vi "TestTranslateVI.vi"(8 "error in (no error)":errorcluster) -> (0 "error out":errorcluster)   [LabVIEW 2017]
uses:
  <vilib>/addons/_JKI Toolkits/Caraya/classes/Test/Test.lvclass
  src/API/JKI Simple Localization.lvlib
  <vilib>/addons/_JKI Toolkits/Caraya/classes/Assert/Assert.lvclass
panel:
  # "See block diagram for unit tests of TranslateVI.vi"
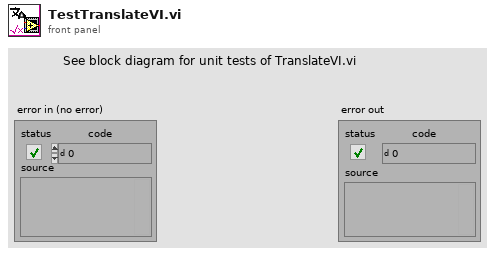
[diagram p1: front panel]
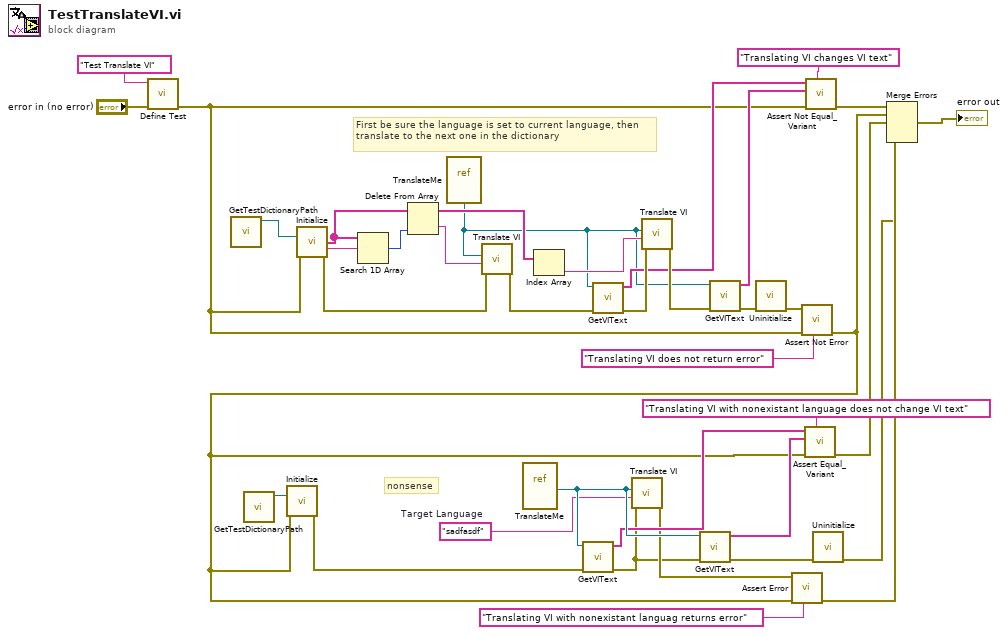
[diagram p0: block diagram]
diagram:
  w22 = "sadfasdf"  # Target Language
  # "nonsense"
  # "First be sure the language is set to current language, then translate to the next one in the dictionary"
  n1 = call <vilib>:"Define Test.vi"("error in (no error)"="error in (no error)", "Label (VI Title)"="Test Translate VI") -> ("error out"=w19:errorcluster)  [unwired: 9 in]
  n2 = call "GetTestDictionaryPath.vi"() -> ("Test Dictionary Path"=w36:path)  [unwired: 11 in]
  n3 = call "GetTestDictionaryPath.vi"() -> ("Test Dictionary Path"=w21:path)  [unwired: 11 in]
  n4 = call "Initialize.vi"("Dictionary File Path"=w36, "error in"=w19) -> ("Languages"=w30:string[], "Current Language"=w11:string, "error out"=w8:errorcluster)  [unwired: 10 in, 1 out]
  n5 = Search 1D Array(1D array=w30, element=w11) -> (index of element=w31:i32)  [unwired: 1 in]
  n6 = Delete From Array(array=w30, index=w31) -> (deleted portion=w9:string, array with subset deleted=w13:string[])  [unwired: 1 in]
  n7 = vi-ref "TranslateMe.vi"() -> (w10:refnum<vi>)
  n8 = call "Translate VI.vi"("error in"=w8, "Target Language"=w9, "VI Ref"=w10) -> ("error out"=w7:errorcluster)  [unwired: 8 in]
  n9 = vi-ref "TranslateMe.vi"() -> (w24:refnum<vi>)
  n10 = Index Array(array=w13) -> (element=w12:string)  [unwired: 1 in]
  n11 = call "GetVIText.vi"("error in (no error)"=w7, "VI"=w10) -> ("error out"=w29:errorcluster, "Control Text"=w26:string[])  [unwired: 7 in, 1 out]
  n12 = call "Translate VI.vi"("error in"=w29, "Target Language"=w12, "VI Ref"=w10) -> ("error out"=w28:errorcluster)  [unwired: 8 in]
  n13 = call "GetVIText.vi"("error in (no error)"=w28, "VI"=w10) -> ("error out"=w27:errorcluster, "Control Text"=w25:string[])  [unwired: 7 in, 1 out]
  n14 = call "Uninitialize.vi"("error in"=w27) -> ("error out"=w2:errorcluster)  [unwired: 10 in]
  n15 = call <vilib>:"Assert Not Error.vi"("Label"="Translating VI does not return error", "error in (no error)"=w19, "Not Error?"=w2) -> ("error out"=w16:errorcluster)  [unwired: 8 in]
  n16 = call "Initialize.vi"("Dictionary File Path"=w21, "error in"=w16) -> ("error out"=w23:errorcluster)  [unwired: 10 in, 3 out]
  n17 = call "GetVIText.vi"("error in (no error)"=w23, "VI"=w24) -> ("error out"=w5:errorcluster, "Control Text"=w17:string[])  [unwired: 7 in, 1 out]
  n18 = call "Translate VI.vi"("error in"=w5, "Target Language"=w22, "VI Ref"=w24) -> ("error out"=w6:errorcluster)  [unwired: 8 in]
  n19 = call "GetVIText.vi"("error in (no error)"=w5, "VI"=w24) -> ("error out"=w4:errorcluster, "Control Text"=w18:string[])  [unwired: 7 in, 1 out]
  n20 = call <vilib>:"Assert Error.vi"("Label"="Translating VI with nonexistant languag returns error", "error in (no error)"=w16, "Error?"=w6) -> ("error out"=w3:errorcluster)  [unwired: 8 in]
  n21 = call <vilib>:"Assert Equal_Variant.vi"("Label"="Translating VI with nonexistant language does not change VI text", "error in (no error)"=w16, "Y"=w18, "X"=w17) -> ("error out"=w14:errorcluster)  [unwired: 7 in]
  n22 = call <vilib>:"Assert Not Equal_Variant.vi"("Label"="Translating VI changes VI text", "error in (no error)"=w19, "Y"=w25, "X"=w26) -> ("error out"=w34:errorcluster)  [unwired: 7 in]
  n23 = call "Uninitialize.vi"("error in"=w4) -> ("error out"=w1:errorcluster)  [unwired: 10 in]
  n24 = Merge Errors(w34, w16, w14, w1, w3) -> (→"error out":errorcluster)
